vi "UPRcontroller_v00_basedonlsmv66.vi"() -> ()   [LabVIEW 2015] (continued)
                        n4652 = local read "Vx-ref"() -> (w1526:dbl)
                        n4653 = local read "Vy-ref"() -> (w1528:dbl)
                        n4654 = local read "avpp"() -> (w1527:i32)
                        n4655 = call "tt_timeandsamples.vi"("bin"=w1521, "refreshtime"=w1515, "srateAODOtt"=w1518, "tot#ofsamples"=w1523) -> ("refreshrate"=w1519:dbl, "refreshbuffer"=w1520:i32, "timetracecycles"=w1525:i32)  [unwired: 5 in]
                        n4656 = local read "bin"() -> (w1522:dbl)
                        n4657 = call "2pparameters.vi"("command"="get") -> ("params out"=w1534:T12)  [unwired: 1 in]
                        n4658 = Bundle By Name(cluster=w1534, "Drawing Mode"=w1507, "measpoints"=w1523, "tt_cycles"=w1525, "refreshbuffer"=w1520, "refreshrate"=w1519, "Vx-ref"=w1526, "Vy-ref"=w1528, "srate"=w1517, "finite"=w1530, "cont"=w1529, "wavdet"=w1531, "avpp"=w1527, "srateAODO"=w1524, "bufferAI"=w1520, "bin"=w1522, "Angle Img"=w1514, "Vxminref"=w1513, "Vxmaxref"=w1512, "Vyminref"=w1511, "Vymaxref"=w1510, "Xpixels Img"=w1509, "Ypixels Img"=w1508, "Pel"=w1506, "Vz-reset"=0.0, "AIoverride"=w1504, "type"="Timetrace") -> (w1532:T12)
                        n4659 = Reciprocal(x=w1519) -> (1/x=w1516:dbl)
                        n4660 = local write "refreshtime"(w1516) -> ()
                        n4661 = call "2pparameters.vi"("Params in"=w1532, "command"="set") -> ()  [unwired: 1 out]
                      }
                      frame "Lifetime (point)" {
                      }
                    }
                  }
                  frame #1 {
                    w1537 = FALSE ("wavdet")
                    n4662 = call "2pparameters.vi"("command"="get") -> ("params out"=w1541:T12)  [unwired: 1 in]
                    n4663 = Bundle By Name(cluster=w1541, "finite"=w1537, "cont"=w1537, "wavdet"=TRUE) -> (w1538:T12)
                    n4664 = call "2pparameters.vi"("Params in"=w1538, "command"="set") -> ()  [unwired: 1 out]
                  }
                  frame #2 {
                    n4665 = local read "Meastab"() -> (w1568:enum32{"X-Y Image", "Linescan", "Timetrace"})
                    n4666 = property on="AO channels" class="Ring (strict)"() -> ("RingText.Text"=w1543:string)  [unwired: 2 in, 2 out]
                    n4667 = property on="refwf" class="Ring (strict)"() -> ("RingText.Text"=w1567:string)  [unwired: 2 in, 2 out]
                    n4668 = local read "Build analog waveform tabs"() -> (w1566:enum32{"Square", "Triangle", "Matlab"})
                    n4669 = case shown="\"X-Y Image\", Default" w1568 {
                      tunnel: [w1574 w1575] -> w1565
                      frame "X-Y Image", Default {
                        n4670 = local read "Sampling rate"() -> (w1574:dbl)
                      }
                      frame "Timetrace" {
                        n4671 = local read "srateAODOtt"() -> (w1575:dbl)
                      }
                    }
                    n4672 = local read "Matlab waveform path"() -> (w1558:path)
                    n4673 = local read "Period (ms)"() -> (w1561:dbl)
                    n4674 = local read "Frequency"() -> (w1560:dbl)
                    n4675 = local read "Tri Repeats"() -> (w1559:dbl)
                    n4676 = local read "Repeats"() -> (w1564:dbl)
                    n4677 = local read "Cycles"() -> (w1563:dbl)
                    n4678 = local read "Pulses"() -> (w1562:dbl)
                    n4679 = call "matlabwfexistsdialogue.vi"("Matlab waveform path"=w1558) -> ("mtalab waveform path out"=w1557:path)
                    n4680 = call "wfsizecalc.vi"("Sampling frequency (Hz)"=w1565, "AOtab"=w1566, "reference waveforms to"=w1567, "channel"=w1543, "Repeats"=w1564, "Cycles"=w1563, "Matlab wave file"=w1557, "pulses"=w1562, "Period (ms)"=w1561, "Frequency"=w1560, "Tri Repeats"=w1559) -> ("total size GB"=w1552:dbl, "gigabytesize wf"=w1548:dbl)  [unwired: 3 in]
                    n4681 = Greater?(x=w1548, y=0.5) -> (0:w1549:bool)
                    n4682 = Number To Fractional String(number=w1548, width (-)=i16 3) -> (F-format string=w1554:string)  [unwired: 2 in]
                    n4683 = Number To Fractional String(number=w1552, width (-)=i16 4) -> (F-format string=w1553:string)  [unwired: 2 in]
                    n4684 = Concatenate Strings("this is a crude approximation:\nyou're about to create a  " ("message"), w1554, " GB waveform for a total of " ("string"), w1553, " GB. Are you sure?" ("string")) -> (w1550:string)
                    n4685 = case shown="True" w1549 {
                      tunnel: w1550 -> [_ w1573]
                      tunnel: [TRUE ("T button?") w1570] -> w1544
                      frame False {
                      }
                      frame True {
                        n4686 = Two Button Dialog(message=w1573, 1:"No, don't do this." ("Center Button Text (\"No\")"), 2:"Yes, continue. " ("Left Button Text (\"Yes\")")) -> (T button?=w1570:bool)
                      }
                    }
                  }
                  frame #3 {
                    n4687 = case shown="True" w1576 {
                      tunnel: [_ w1580] -> w1578
                      tunnel: [_ w1579] -> w1577
                      frame False {
                      }
                      frame True {
                        n4688 = local read "AO channels"() -> (w1582:u32)
                        n4689 = call "2pparameters.vi"("command"="get") -> ("params out"=w1584:T12)  [unwired: 1 in]
                        n4690 = Unbundle By Name(w1584) -> ("aAO"=w1583:u32[])
                        n4691 = Search 1D Array(1D array=w1583, element=w1582) -> (index of element=w1580:i32)  [unwired: 1 in]
                        n4692 = Greater?(x=w1580, y=-1) -> (0:w1579:bool)
                        n4693 = case shown="True" w1579 {
                          tunnel: w1580 -> [_ w1594]
                          frame False {
                          }
                          frame True {
                            n4694 = local read "Meastab"() -> (w1587:enum32{"X-Y Image", "Linescan", "Timetrace"})
                            n4695 = local read "Tri padding value"() -> (w1588:dbl)
                            n4696 = local read "Amplitude (V)"() -> (w1592:dbl)
                            n4697 = local read "Tri Phase (s)"() -> (w1589:dbl)
                            n4698 = local read "Tri Repeats"() -> (w1590:dbl)
                            n4699 = local read "Frequency"() -> (w1591:dbl)
                            n4700 = local read "Offset (V)"() -> (w1593:dbl)
                            n4701 = case shown="\"Timetrace\"" w1587 {
                              tunnel: [w1595 w1596] -> w1586
                              frame "X-Y Image", Default {
                                n4702 = local read "Sampling rate"() -> (w1595:dbl)
                              }
                              frame "Timetrace" {
                                n4703 = local read "srateAODOtt"() -> (w1596:dbl)
                              }
                            }
                            n4704 = call "replace AO tri wf param.vi"("padding value"=w1588, "index of AO wave"=w1594, "Tri phase"=w1589, "Sampling frequency (Hz)"=w1586, "Tri Repeats"=w1590, "Frequency"=w1591, "Amplitude (V)"=w1592, "Offset (V)"=w1593) -> ()
                          }
                        }
                      }
                    }
                  }
                  frame #4 {
                    n4705 = case shown="True" w1597 {
                      tunnel: w1599 -> [_ w1601]
                      tunnel: w1598 -> [_ w1600]
                      frame False {
                      }
                      frame True {
                        n4706 = case shown="True" w1600 {
                          tunnel: w1601 -> [_ w1610]
                          frame False {
                          }
                          frame True {
                            n4707 = call "waveformparamsv2.vi"("command"="get") -> ("Params out"=w1623:T17)  [unwired: 4 in, 2 out]
                            n4708 = Unbundle By Name(w1623) -> ("AO parameters"=w1622:T18)
                            n4709 = local read "Meastab"() -> (w1605:enum32{"X-Y Image", "Linescan", "Timetrace"})
                            n4710 = case shown="\"Timetrace\"" w1605 {
                              tunnel: [w1625 w1626] -> w1604
                              frame "X-Y Image", Default {
                                n4711 = local read "Sampling rate"() -> (w1625:dbl)
                              }
                              frame "Timetrace" {
                                n4712 = local read "srateAODOtt"() -> (w1626:dbl)
                              }
                            }
                            n4713 = Index Array(array=w1622, index=w1610) -> (element=w1612:T19)
                            n4714 = call "waveformsAObuffer.vi"("command"="get") -> ("AO wf out"=w1611:waveform(dbl)[])  [unwired: 1 in]
                            n4715 = call "generateTriWave_fromAOparameters.vi"("AO params"=w1612) -> ("Waveform"=w1609:waveform(dbl))  [unwired: 1 out]
                            n4716 = property on="refwf" class="Ring (strict)"() -> ("RingText.Text"=w1613:string)  [unwired: 2 in, 2 out]
                            n4717 = Replace Array Subset(array=w1611, new element=w1609, index=w1610) -> (w1608:waveform(dbl)[])
                            n4718 = call "waveformsDObuffer.vi"("command"="get") -> ("DO wf out"=w1618:digitalwaveform[])  [unwired: 1 in]
                            n4719 = call "correctwaveformsizetemp.vi"("new sampling frequency (Hz)"=w1604, "start"=FALSE, "reference waveforms to"=w1613, "Analog waveforms in"=w1608, "stop"=FALSE, "Digital waveforms in"=w1618) -> ("analog wf out"=w1616:waveform(dbl)[], "Digital wf out"=w1614:digitalwaveform[], "measpoints"=w1606:i32)
                            n4720 = local read "wavdet"() -> (w1607:bool)
                            n4721 = local write "Analog Lines Plot"(w1616) -> ()
                            n4722 = call "GetNumCamFramesv2.vi"("Digital Waveform Graph"=w1614) -> ("Numeric"=w1615:i32)  [unwired: 10 in]
                            n4723 = local write "Digital Lines Plot"(w1614) -> ()
                            n4724 = call "waveformsAObuffer.vi"("AO wf in"=w1616, "command"="set") -> ()  [unwired: 1 out]
                            n4725 = call "waveformsDObuffer.vi"("DO wf in"=w1614, "command"="set") -> ()  [unwired: 1 out]
                            n4726 = local write "Total Camera Frames"(w1615) -> ()
                            n4727 = case shown="True" w1607 {
                              tunnel: w1606 -> [_ w1627]
                              frame False {
                              }
                              frame True {
                                n4728 = local write "# of frames"(w1627) -> ()
                              }
                            }
                          }
                        }
                      }
                    }
                  }
                  frame #5 {
                    w1629 = FALSE ("addAO")
                    n4729 = case shown="True" w1628 {
                      frame False {
                      }
                      frame True {
                        n4730 = local write "not loadedtri"(FALSE ("not loadedtri")) -> ()
                      }
                    }
                    n4731 = local write "changeAOtri"(w1629) -> ()
                    n4732 = property on="load changed AOtri" class="Bool (strict)"("Val(Sgnl)"=w1629) -> ()  [unwired: 2 in, 2 out]
                    n4733 = local read "finite samples"() -> (w1630:bool)
                    n4734 = local read "continuous"() -> (w1631:bool)
                    n4735 = local read "wavdet"() -> (w1632:bool)
                    n4736 = call "2pparameters.vi"("command"="get") -> ("params out"=w1635:T12)  [unwired: 1 in]
                    n4737 = Bundle By Name(cluster=w1635, "finite"=w1630, "cont"=w1631, "wavdet"=w1632) -> (w1633:T12)
                    n4738 = call "2pparameters.vi"("Params in"=w1633, "command"="set") -> ()  [unwired: 1 out]
                  }
                }
              }
            }
          }
          event "Load Matlab Waveform": Value Change {
            n4739 = event-data() -> ("NewVal"=w1638:bool)  [unwired: 1 in, 5 out]
            n4740 = case shown="True" w1638 {
              frame False {
              }
              frame True {
                n4741 = stacked-sequence {
                  seq-local: [_ _ _ w1780 _ _] -> [_ _ _ _ w1798 _]
                  seq-local: [_ _ _ w1779 _ _] -> [_ _ _ _ w1797 _]
                  seq-local: [_ _ w1746 _ _ _] -> [_ _ _ w1778 w1796 w1827]
                  frame #0 {
                    n4742 = local read "Measurement"() -> (w1640:T4)
                    n4743 = case shown="\"X-Y-t movie\", Default" w1640 {
                      frame "X-Y-t movie", Default {
                        n4744 = local read "avpp"() -> (w1661:i32)
                        n4745 = local read "Angle ref"() -> (w1660:dbl)
                        n4746 = local read "ROI Type"() -> (w1659:u16)
                        n4747 = local read "xpixels ref"() -> (w1656:i32)
                        n4748 = local read "Vx-min ref"() -> (w1655:dbl)
                        n4749 = local read "Vx-max ref"() -> (w1654:dbl)
                        n4750 = local read "ypixels ref"() -> (w1652:i32)
                        n4751 = local read "Vy-min ref"() -> (w1653:dbl)
                        n4752 = local read "Vy-max ref"() -> (w1649:dbl)
                        n4753 = local read "Sampling rate"() -> (w1643:dbl)
                        n4754 = local read "finite samples"() -> (w1644:bool)
                        n4755 = local read "continuous"() -> (w1647:bool)
                        n4756 = local read "wavdet"() -> (w1648:bool)
                        n4757 = local read "# of frames"() -> (w1646:i32)
                        n4758 = local read "maxbufferAI"() -> (w1645:i32)
                        n4759 = local read "Override AI buffer"() -> (w1641:bool)
                        n4760 = call "2pparameters.vi"("command"="get") -> ("params out"=w1658:T12)  [unwired: 1 in]
                        n4761 = Bundle By Name(cluster=w1658, "type"="X-Y-t movie", "avpp"=w1661, "Angle Img"=w1660, "Xpixels Img"=w1656, "Vx-min Img"=w1655, "VX-max Img"=w1654, "Ypixels Img"=w1652, "Vy-min Img"=w1653, "Vy-max Img"=w1649, "srate"=w1643, "srate Img"=w1643, "finite"=w1644, "cont"=w1647, "wavdet"=w1648, "measpoints"=w1646, "maxbufferAI"=w1645, "Drawing Mode"=w1659, "Vz-reset"=0.0, "AIoverride"=w1641) -> (w1650:T12)
                        n4762 = call "2pparameters.vi"("Params in"=w1650, "command"="set") -> ()  [unwired: 1 out]
                      }
                      frame "X-Y-Z stack" {
                        n4763 = call "2pparameters.vi"("command"="get") -> ("params out"=w1665:T12)  [unwired: 1 in]
                        n4764 = Bundle By Name(cluster=w1665, "type"="X-Y-Z stack") -> (w1663:T12)
                        n4765 = call "2pparameters.vi"("Params in"=w1663, "command"="set") -> ()  [unwired: 1 out]
                      }
                      frame "Lifetime (scan)" {
                        n4766 = call "2pparameters.vi"("command"="get") -> ("params out"=w1670:T12)  [unwired: 1 in]
                        n4767 = Bundle By Name(cluster=w1670, "type"="Lifetime (scan)") -> (w1668:T12)
                        n4768 = call "2pparameters.vi"("Params in"=w1668, "command"="set") -> ()  [unwired: 1 out]
                      }
                      frame "Lifetime (contour)" {
                        n4769 = local read "Vy-min draw"() -> (w1680:dbl)
                        n4770 = local read "Vy-max draw"() -> (w1679:dbl)
                        n4771 = local read "Vx-min draw"() -> (w1682:dbl)
                        n4772 = local read "Vx-max draw"() -> (w1681:dbl)
                        n4773 = local read "xpixels ref"() -> (w1678:i32)
                        n4774 = local read "ypixels ref"() -> (w1677:i32)
                        n4775 = local read "ROI Type"() -> (w1676:u16)
                        n4776 = local read "srateAODOtt"() -> (w1687:dbl)
                        n4777 = local read "# of frames"() -> (w1692:i32)
                        n4778 = local read "refreshtime"() -> (w1684:dbl)
                        n4779 = local read "Pel"() -> (w1675:dbl)
                        n4780 = local read "bin"() -> (w1690:dbl)
                        n4781 = local read "Override AI buffer"() -> (w1673:bool)
                        n4782 = local read "finite samples"() -> (w1699:bool)
                        n4783 = local read "srateAODOtt"() -> (w1686:dbl)
                        n4784 = local read "srateAODOtt"() -> (w1693:dbl)
                        n4785 = local read "continuous"() -> (w1698:bool)
                        n4786 = local read "Angle ref"() -> (w1683:dbl)
                        n4787 = local read "wavdet"() -> (w1700:bool)
                        n4788 = local read "Vx-ref"() -> (w1695:dbl)
                        n4789 = local read "Vy-ref"() -> (w1697:dbl)
                        n4790 = local read "avpp"() -> (w1696:i32)
                        n4791 = call "tt_timeandsamples.vi"("bin"=w1690, "refreshtime"=w1684, "srateAODOtt"=w1687, "tot#ofsamples"=w1692) -> ("refreshrate"=w1688:dbl, "refreshbuffer"=w1689:i32, "timetracecycles"=w1694:i32)  [unwired: 5 in]
                        n4792 = local read "bin"() -> (w1691:dbl)
                        n4793 = call "2pparameters.vi"("command"="get") -> ("params out"=w1703:T12)  [unwired: 1 in]
                        n4794 = Bundle By Name(cluster=w1703, "Drawing Mode"=w1676, "measpoints"=w1692, "tt_cycles"=w1694, "refreshbuffer"=w1689, "refreshrate"=w1688, "Vx-ref"=w1695, "Vy-ref"=w1697, "srate"=w1686, "finite"=w1699, "cont"=w1698, "wavdet"=w1700, "avpp"=w1696, "srateAODO"=w1693, "bufferAI"=w1689, "bin"=w1691, "Angle Img"=w1683, "Vxminref"=w1682, "Vxmaxref"=w1681, "Vyminref"=w1680, "Vymaxref"=w1679, "Xpixels Img"=w1678, "Ypixels Img"=w1677, "Pel"=w1675, "Vz-reset"=0.0, "AIoverride"=w1673, "type"="Lifetime (contour)") -> (w1701:T12)
                        n4795 = Reciprocal(x=w1688) -> (1/x=w1685:dbl)
                        n4796 = local write "refreshtime"(w1685) -> ()
                        n4797 = call "2pparameters.vi"("Params in"=w1701, "command"="set") -> ()  [unwired: 1 out]
                      }
                      frame "X-Y-Z-t movie" {
                      }
                      frame "linescan" {
                      }
                      frame "Timetrace" {
                        n4798 = local read "Vy-min draw"() -> (w1713:dbl)
                        n4799 = local read "Vy-max draw"() -> (w1712:dbl)
                        n4800 = local read "Vx-min draw"() -> (w1715:dbl)
                        n4801 = local read "Vx-max draw"() -> (w1714:dbl)
                        n4802 = local read "xpixels ref"() -> (w1711:i32)
                        n4803 = local read "ypixels ref"() -> (w1710:i32)
                        n4804 = local read "ROI Type"() -> (w1709:u16)
                        n4805 = local read "srateAODOtt"() -> (w1720:dbl)
                        n4806 = local read "# of frames"() -> (w1725:i32)
                        n4807 = local read "refreshtime"() -> (w1717:dbl)
                        n4808 = local read "Pel"() -> (w1708:dbl)
                        n4809 = local read "bin"() -> (w1723:dbl)
                        n4810 = local read "Override AI buffer"() -> (w1706:bool)
                        n4811 = local read "finite samples"() -> (w1732:bool)
                        n4812 = local read "srateAODOtt"() -> (w1719:dbl)
                        n4813 = local read "srateAODOtt"() -> (w1726:dbl)
                        n4814 = local read "continuous"() -> (w1731:bool)
                        n4815 = local read "Angle ref"() -> (w1716:dbl)
                        n4816 = local read "wavdet"() -> (w1733:bool)
                        n4817 = local read "Vx-ref"() -> (w1728:dbl)
                        n4818 = local read "Vy-ref"() -> (w1730:dbl)
                        n4819 = local read "avpp"() -> (w1729:i32)
                        n4820 = call "tt_timeandsamples.vi"("bin"=w1723, "refreshtime"=w1717, "srateAODOtt"=w1720, "tot#ofsamples"=w1725) -> ("refreshrate"=w1721:dbl, "refreshbuffer"=w1722:i32, "timetracecycles"=w1727:i32)  [unwired: 5 in]
                        n4821 = local read "bin"() -> (w1724:dbl)
                        n4822 = call "2pparameters.vi"("command"="get") -> ("params out"=w1736:T12)  [unwired: 1 in]
                        n4823 = Bundle By Name(cluster=w1736, "Drawing Mode"=w1709, "measpoints"=w1725, "tt_cycles"=w1727, "refreshbuffer"=w1722, "refreshrate"=w1721, "Vx-ref"=w1728, "Vy-ref"=w1730, "srate"=w1719, "finite"=w1732, "cont"=w1731, "wavdet"=w1733, "avpp"=w1729, "srateAODO"=w1726, "bufferAI"=w1722, "bin"=w1724, "Angle Img"=w1716, "Vxminref"=w1715, "Vxmaxref"=w1714, "Vyminref"=w1713, "Vymaxref"=w1712, "Xpixels Img"=w1711, "Ypixels Img"=w1710, "Pel"=w1708, "Vz-reset"=0.0, "AIoverride"=w1706, "type"="Timetrace") -> (w1734:T12)
                        n4824 = Reciprocal(x=w1721) -> (1/x=w1718:dbl)
                        n4825 = local write "refreshtime"(w1718) -> ()
                        n4826 = call "2pparameters.vi"("Params in"=w1734, "command"="set") -> ()  [unwired: 1 out]
                      }
                      frame "Lifetime (point)" {
                      }
                    }
                    n4827 = local write "changeAOmatlab"(TRUE ("addAO")) -> ()
                  }
                  frame #1 {
                    w1739 = FALSE ("wavdet")
                    n4828 = call "2pparameters.vi"("command"="get") -> ("params out"=w1743:T12)  [unwired: 1 in]
                    n4829 = Bundle By Name(cluster=w1743, "finite"=w1739, "cont"=w1739, "wavdet"=TRUE) -> (w1740:T12)
                    n4830 = call "2pparameters.vi"("Params in"=w1740, "command"="set") -> ()  [unwired: 1 out]
                  }
                  frame #2 {
                    n4831 = local read "Meastab"() -> (w1770:enum32{"X-Y Image", "Linescan", "Timetrace"})
                    n4832 = property on="AO channels" class="Ring (strict)"() -> ("RingText.Text"=w1745:string)  [unwired: 2 in, 2 out]
                    n4833 = property on="refwf" class="Ring (strict)"() -> ("RingText.Text"=w1769:string)  [unwired: 2 in, 2 out]
                    n4834 = local read "Build analog waveform tabs"() -> (w1768:enum32{"Square", "Triangle", "Matlab"})
                    n4835 = case shown="\"X-Y Image\", Default" w1770 {
                      tunnel: [w1776 w1777] -> w1767
                      frame "X-Y Image", Default {
                        n4836 = local read "Sampling rate"() -> (w1776:dbl)
                      }
                      frame "Timetrace" {
                        n4837 = local read "srateAODOtt"() -> (w1777:dbl)
                      }
                    }
                    n4838 = local read "Matlab waveform path"() -> (w1760:path)
                    n4839 = local read "Period (ms)"() -> (w1763:dbl)
                    n4840 = local read "Frequency"() -> (w1762:dbl)
                    n4841 = local read "Tri Repeats"() -> (w1761:dbl)
                    n4842 = local read "Repeats"() -> (w1766:dbl)
                    n4843 = local read "Cycles"() -> (w1765:dbl)
                    n4844 = local read "Pulses"() -> (w1764:dbl)
                    n4845 = call "matlabwfexistsdialogue.vi"("Matlab waveform path"=w1760) -> ("mtalab waveform path out"=w1759:path)
                    n4846 = call "wfsizecalc.vi"("Sampling frequency (Hz)"=w1767, "AOtab"=w1768, "reference waveforms to"=w1769, "channel"=w1745, "Repeats"=w1766, "Cycles"=w1765, "Matlab wave file"=w1759, "pulses"=w1764, "Period (ms)"=w1763, "Frequency"=w1762, "Tri Repeats"=w1761) -> ("total size GB"=w1754:dbl, "gigabytesize wf"=w1750:dbl)  [unwired: 3 in]
                    n4847 = Greater?(x=w1750, y=0.5) -> (0:w1751:bool)
                    n4848 = Number To Fractional String(number=w1750, width (-)=i16 3) -> (F-format string=w1756:string)  [unwired: 2 in]
                    n4849 = Number To Fractional String(number=w1754, width (-)=i16 4) -> (F-format string=w1755:string)  [unwired: 2 in]
                    n4850 = Concatenate Strings("this is a crude approximation:\nyou're about to create a  " ("message"), w1756, " GB waveform for a total of " ("string"), w1755, " GB. Are you sure?" ("string")) -> (w1752:string)
                    n4851 = case shown="True" w1751 {
                      tunnel: w1752 -> [_ w1775]
                      tunnel: [TRUE ("T button?") w1772] -> w1746
                      frame False {
                      }
                      frame True {
                        n4852 = Two Button Dialog(message=w1775, 1:"No, don't do this." ("Center Button Text (\"No\")"), 2:"Yes, continue. " ("Left Button Text (\"Yes\")")) -> (T button?=w1772:bool)
                      }
                    }
                  }
                  frame #3 {
                    n4853 = case shown="True" w1778 {
                      tunnel: [_ w1782] -> w1780
                      tunnel: [_ w1781] -> w1779
                      frame False {
                      }
                      frame True {
                        n4854 = local read "AO channels"() -> (w1784:u32)
                        n4855 = call "2pparameters.vi"("command"="get") -> ("params out"=w1786:T12)  [unwired: 1 in]
                        n4856 = Unbundle By Name(w1786) -> ("aAO"=w1785:u32[])
                        n4857 = Search 1D Array(1D array=w1785, element=w1784) -> (index of element=w1782:i32)  [unwired: 1 in]
                        n4858 = Greater?(x=w1782, y=-1) -> (0:w1781:bool)
                        n4859 = case shown="True" w1781 {
                          tunnel: w1782 -> [_ w1793]
                          frame False {
                          }
                          frame True {
                            n4860 = local read "Meastab"() -> (w1789:enum32{"X-Y Image", "Linescan", "Timetrace"})
                            n4861 = local read "Matlab waveform path"() -> (w1791:path)
                            n4862 = local read "Matlab padding value"() -> (w1792:dbl)
                            n4863 = case shown="\"Timetrace\"" w1789 {
                              tunnel: [w1794 w1795] -> w1788
                              frame "X-Y Image", Default {
                                n4864 = local read "Sampling rate"() -> (w1794:dbl)
                              }
                              frame "Timetrace" {
                                n4865 = local read "srateAODOtt"() -> (w1795:dbl)
                              }
                            }
                            n4866 = call "matlabwfexistsdialogue.vi"("Matlab waveform path"=w1791) -> ("mtalab waveform path out"=w1790:path)
                            n4867 = call "replace AO matlab param.vi"("Sampling frequency (Hz)"=w1788, "matlab wave file"=w1790, "index of AO wave"=w1793, "padding value"=w1792) -> ()  [unwired: 7 in]
                          }
                        }
                      }
                    }
                  }
                  frame #4 {
                    n4868 = case shown="True" w1796 {
                      tunnel: w1798 -> [_ w1800]
                      tunnel: w1797 -> [_ w1799]
                      frame False {
                      }
                      frame True {
                        n4869 = case shown="True" w1799 {
                          tunnel: w1800 -> [_ w1807]
                          frame False {
                          }
                          frame True {
                            n4870 = local read "Meastab"() -> (w1804:enum32{"X-Y Image", "Linescan", "Timetrace"})
                            n4871 = call "waveformparamsv2.vi"("command"="get") -> ("Params out"=w1810:T17)  [unwired: 4 in, 2 out]
                            n4872 = Unbundle By Name(w1810) -> ("AO parameters"=w1809:T18)
                            n4873 = case shown="\"Timetrace\"" w1804 {
                              tunnel: [w1824 w1825] -> w1803
                              frame "X-Y Image", Default {
                                n4874 = local read "Sampling rate"() -> (w1824:dbl)
                              }
                              frame "Timetrace" {
                                n4875 = local read "srateAODOtt"() -> (w1825:dbl)
                              }
                            }
                            n4876 = Index Array(array=w1809, index=w1807) -> (element=w1808:T19)
                            n4877 = call "waveformsAObuffer.vi"("command"="get") -> ("AO wf out"=w1814:waveform(dbl)[])  [unwired: 1 in]
                            n4878 = call "matlabAOwffromparam.vi"("Cluster"=w1808) -> ("Waveform"=w1812:waveform(dbl))  [unwired: 1 out]
                            n4879 = property on="refwf" class="Ring (strict)"() -> ("RingText.Text"=w1815:string)  [unwired: 2 in, 2 out]
                            n4880 = Replace Array Subset(array=w1814, new element=w1812, index=w1807) -> (w1813:waveform(dbl)[])
                            n4881 = call "waveformsDObuffer.vi"("command"="get") -> ("DO wf out"=w1820:digitalwaveform[])  [unwired: 1 in]
                            n4882 = call "correctwaveformsizetemp.vi"("new sampling frequency (Hz)"=w1803, "start"=FALSE, "reference waveforms to"=w1815, "Analog waveforms in"=w1813, "stop"=FALSE, "Digital waveforms in"=w1820) -> ("analog wf out"=w1818:waveform(dbl)[], "Digital wf out"=w1816:digitalwaveform[], "measpoints"=w1805:i32)
                            n4883 = local read "wavdet"() -> (w1806:bool)
                            n4884 = local write "Analog Lines Plot"(w1818) -> ()
                            n4885 = call "GetNumCamFramesv2.vi"("Digital Waveform Graph"=w1816) -> ("Numeric"=w1817:i32)  [unwired: 10 in]
                            n4886 = local write "Digital Lines Plot"(w1816) -> ()
                            n4887 = call "waveformsAObuffer.vi"("AO wf in"=w1818, "command"="set") -> ()  [unwired: 1 out]
                            n4888 = call "waveformsDObuffer.vi"("DO wf in"=w1816, "command"="set") -> ()  [unwired: 1 out]
                            n4889 = local write "Total Camera Frames"(w1817) -> ()
                            n4890 = case shown="True" w1806 {
                              tunnel: w1805 -> [_ w1826]
                              frame False {
                              }
                              frame True {
                                n4891 = local write "# of frames"(w1826) -> ()
                              }
                            }
                          }
                        }
                      }
                    }
                  }
                  frame #5 {
                    w1828 = FALSE ("addAO")
                    n4892 = case shown="True" w1827 {
                      frame False {
                      }
                      frame True {
                        n4893 = local write "not loadedml"(FALSE ("not loadedml")) -> ()
                      }
                    }
                    n4894 = local read "finite samples"() -> (w1829:bool)
                    n4895 = local read "continuous"() -> (w1830:bool)
                    n4896 = local read "wavdet"() -> (w1831:bool)
                    n4897 = property on="Load Matlab Waveform" class="Bool (strict)"("Val(Sgnl)"=w1828) -> ()  [unwired: 2 in, 2 out]
                    n4898 = local write "changeAOmatlab"(w1828) -> ()
                    n4899 = call "2pparameters.vi"("command"="get") -> ("params out"=w1834:T12)  [unwired: 1 in]
                    n4900 = Bundle By Name(cluster=w1834, "finite"=w1829, "cont"=w1830, "wavdet"=w1831) -> (w1832:T12)
                    n4901 = call "2pparameters.vi"("Params in"=w1832, "command"="set") -> ()  [unwired: 1 out]
                  }
                }
              }
            }
          }
          event "Load Matlab Waveform DO": Value Change {
            n4902 = event-data() -> ("NewVal"=w1837:bool)  [unwired: 1 in, 5 out]
            n4903 = case shown="True" w1837 {
              frame False {
              }
              frame True {
                n4904 = stacked-sequence {
                  seq-local: [_ _ w1945 _ _] -> [_ _ _ w1960 _]
                  seq-local: [_ _ w1944 _ _] -> [_ _ _ w1959 _]
                  frame #0 {
                    n4905 = local read "Measurement"() -> (w1839:T4)
                    n4906 = case shown="\"X-Y-t movie\", Default" w1839 {
                      frame "X-Y-t movie", Default {
                        n4907 = local read "avpp"() -> (w1860:i32)
                        n4908 = local read "Angle ref"() -> (w1859:dbl)
                        n4909 = local read "ROI Type"() -> (w1858:u16)
                        n4910 = local read "xpixels ref"() -> (w1855:i32)
                        n4911 = local read "Vx-min ref"() -> (w1854:dbl)
                        n4912 = local read "Vx-max ref"() -> (w1853:dbl)
                        n4913 = local read "ypixels ref"() -> (w1851:i32)
                        n4914 = local read "Vy-min ref"() -> (w1852:dbl)
                        n4915 = local read "Vy-max ref"() -> (w1848:dbl)
                        n4916 = local read "Sampling rate"() -> (w1842:dbl)
                        n4917 = local read "finite samples"() -> (w1843:bool)
                        n4918 = local read "continuous"() -> (w1846:bool)
                        n4919 = local read "wavdet"() -> (w1847:bool)
                        n4920 = local read "# of frames"() -> (w1845:i32)
                        n4921 = local read "maxbufferAI"() -> (w1844:i32)
                        n4922 = local read "Override AI buffer"() -> (w1840:bool)
                        n4923 = call "2pparameters.vi"("command"="get") -> ("params out"=w1857:T12)  [unwired: 1 in]
                        n4924 = Bundle By Name(cluster=w1857, "type"="X-Y-t movie", "avpp"=w1860, "Angle Img"=w1859, "Xpixels Img"=w1855, "Vx-min Img"=w1854, "VX-max Img"=w1853, "Ypixels Img"=w1851, "Vy-min Img"=w1852, "Vy-max Img"=w1848, "srate"=w1842, "srate Img"=w1842, "finite"=w1843, "cont"=w1846, "wavdet"=w1847, "measpoints"=w1845, "maxbufferAI"=w1844, "Drawing Mode"=w1858, "Vz-reset"=0.0, "AIoverride"=w1840) -> (w1849:T12)
                        n4925 = call "2pparameters.vi"("Params in"=w1849, "command"="set") -> ()  [unwired: 1 out]
                      }
                      frame "X-Y-Z stack" {
                        n4926 = call "2pparameters.vi"("command"="get") -> ("params out"=w1864:T12)  [unwired: 1 in]
                        n4927 = Bundle By Name(cluster=w1864, "type"="X-Y-Z stack") -> (w1862:T12)
                        n4928 = call "2pparameters.vi"("Params in"=w1862, "command"="set") -> ()  [unwired: 1 out]
                      }
                      frame "Lifetime (scan)" {
                        n4929 = call "2pparameters.vi"("command"="get") -> ("params out"=w1869:T12)  [unwired: 1 in]
                        n4930 = Bundle By Name(cluster=w1869, "type"="Lifetime (scan)") -> (w1867:T12)
                        n4931 = call "2pparameters.vi"("Params in"=w1867, "command"="set") -> ()  [unwired: 1 out]
                      }
                      frame "Lifetime (contour)" {
                        n4932 = local read "Vy-min draw"() -> (w1879:dbl)
                        n4933 = local read "Vy-max draw"() -> (w1878:dbl)
                        n4934 = local read "Vx-min draw"() -> (w1881:dbl)
                        n4935 = local read "Vx-max draw"() -> (w1880:dbl)
                        n4936 = local read "xpixels ref"() -> (w1877:i32)
                        n4937 = local read "ypixels ref"() -> (w1876:i32)
                        n4938 = local read "ROI Type"() -> (w1875:u16)
                        n4939 = local read "srateAODOtt"() -> (w1886:dbl)
                        n4940 = local read "# of frames"() -> (w1891:i32)
                        n4941 = local read "refreshtime"() -> (w1883:dbl)
                        n4942 = local read "Pel"() -> (w1874:dbl)
                        n4943 = local read "bin"() -> (w1889:dbl)
                        n4944 = local read "Override AI buffer"() -> (w1872:bool)
                        n4945 = local read "finite samples"() -> (w1898:bool)
                        n4946 = local read "srateAODOtt"() -> (w1885:dbl)
                        n4947 = local read "srateAODOtt"() -> (w1892:dbl)
                        n4948 = local read "continuous"() -> (w1897:bool)
                        n4949 = local read "Angle ref"() -> (w1882:dbl)
                        n4950 = local read "wavdet"() -> (w1899:bool)
                        n4951 = local read "Vx-ref"() -> (w1894:dbl)
                        n4952 = local read "Vy-ref"() -> (w1896:dbl)
                        n4953 = local read "avpp"() -> (w1895:i32)
                        n4954 = call "tt_timeandsamples.vi"("bin"=w1889, "refreshtime"=w1883, "srateAODOtt"=w1886, "tot#ofsamples"=w1891) -> ("refreshrate"=w1887:dbl, "refreshbuffer"=w1888:i32, "timetracecycles"=w1893:i32)  [unwired: 5 in]
                        n4955 = local read "bin"() -> (w1890:dbl)
                        n4956 = call "2pparameters.vi"("command"="get") -> ("params out"=w1902:T12)  [unwired: 1 in]
                        n4957 = Bundle By Name(cluster=w1902, "Drawing Mode"=w1875, "measpoints"=w1891, "tt_cycles"=w1893, "refreshbuffer"=w1888, "refreshrate"=w1887, "Vx-ref"=w1894, "Vy-ref"=w1896, "srate"=w1885, "finite"=w1898, "cont"=w1897, "wavdet"=w1899, "avpp"=w1895, "srateAODO"=w1892, "bufferAI"=w1888, "bin"=w1890, "Angle Img"=w1882, "Vxminref"=w1881, "Vxmaxref"=w1880, "Vyminref"=w1879, "Vymaxref"=w1878, "Xpixels Img"=w1877, "Ypixels Img"=w1876, "Pel"=w1874, "Vz-reset"=0.0, "AIoverride"=w1872, "type"="Lifetime (contour)") -> (w1900:T12)
                        n4958 = Reciprocal(x=w1887) -> (1/x=w1884:dbl)
                        n4959 = local write "refreshtime"(w1884) -> ()
                        n4960 = call "2pparameters.vi"("Params in"=w1900, "command"="set") -> ()  [unwired: 1 out]
                      }
                      frame "X-Y-Z-t movie" {
                      }
                      frame "linescan" {
                      }
                      frame "Timetrace" {
                        n4961 = local read "Vy-min draw"() -> (w1912:dbl)
                        n4962 = local read "Vy-max draw"() -> (w1911:dbl)
                        n4963 = local read "Vx-min draw"() -> (w1914:dbl)
                        n4964 = local read "Vx-max draw"() -> (w1913:dbl)
                        n4965 = local read "xpixels ref"() -> (w1910:i32)
                        n4966 = local read "ypixels ref"() -> (w1909:i32)
                        n4967 = local read "ROI Type"() -> (w1908:u16)
                        n4968 = local read "srateAODOtt"() -> (w1919:dbl)
                        n4969 = local read "# of frames"() -> (w1924:i32)
                        n4970 = local read "refreshtime"() -> (w1916:dbl)
                        n4971 = local read "Pel"() -> (w1907:dbl)
                        n4972 = local read "bin"() -> (w1922:dbl)
                        n4973 = local read "Override AI buffer"() -> (w1905:bool)
                        n4974 = local read "finite samples"() -> (w1931:bool)
                        n4975 = local read "srateAODOtt"() -> (w1918:dbl)
                        n4976 = local read "srateAODOtt"() -> (w1925:dbl)
                        n4977 = local read "continuous"() -> (w1930:bool)
                        n4978 = local read "Angle ref"() -> (w1915:dbl)
                        n4979 = local read "wavdet"() -> (w1932:bool)
                        n4980 = local read "Vx-ref"() -> (w1927:dbl)
                        n4981 = local read "Vy-ref"() -> (w1929:dbl)
                        n4982 = local read "avpp"() -> (w1928:i32)
                        n4983 = call "tt_timeandsamples.vi"("bin"=w1922, "refreshtime"=w1916, "srateAODOtt"=w1919, "tot#ofsamples"=w1924) -> ("refreshrate"=w1920:dbl, "refreshbuffer"=w1921:i32, "timetracecycles"=w1926:i32)  [unwired: 5 in]
                        n4984 = local read "bin"() -> (w1923:dbl)
                        n4985 = call "2pparameters.vi"("command"="get") -> ("params out"=w1935:T12)  [unwired: 1 in]
                        n4986 = Bundle By Name(cluster=w1935, "Drawing Mode"=w1908, "measpoints"=w1924, "tt_cycles"=w1926, "refreshbuffer"=w1921, "refreshrate"=w1920, "Vx-ref"=w1927, "Vy-ref"=w1929, "srate"=w1918, "finite"=w1931, "cont"=w1930, "wavdet"=w1932, "avpp"=w1928, "srateAODO"=w1925, "bufferAI"=w1921, "bin"=w1923, "Angle Img"=w1915, "Vxminref"=w1914, "Vxmaxref"=w1913, "Vyminref"=w1912, "Vymaxref"=w1911, "Xpixels Img"=w1910, "Ypixels Img"=w1909, "Pel"=w1907, "Vz-reset"=0.0, "AIoverride"=w1905, "type"="Timetrace") -> (w1933:T12)
                        n4987 = Reciprocal(x=w1920) -> (1/x=w1917:dbl)
                        n4988 = local write "refreshtime"(w1917) -> ()
                        n4989 = call "2pparameters.vi"("Params in"=w1933, "command"="set") -> ()  [unwired: 1 out]
                      }
                      frame "Lifetime (point)" {
                      }
                    }
                    n4990 = local write "changeDOmatlab"(TRUE ("addAO")) -> ()
                  }
                  frame #1 {
                    w1938 = FALSE ("wavdet")
                    n4991 = call "2pparameters.vi"("command"="get") -> ("params out"=w1942:T12)  [unwired: 1 in]
                    n4992 = Bundle By Name(cluster=w1942, "finite"=w1938, "cont"=w1938, "wavdet"=TRUE) -> (w1939:T12)
                    n4993 = call "2pparameters.vi"("Params in"=w1939, "command"="set") -> ()  [unwired: 1 out]
                  }
                  frame #2 {
                    n4994 = local read "DO channels"() -> (w1947:u16)
                    n4995 = call "2pparameters.vi"("command"="get") -> ("params out"=w1949:T12)  [unwired: 1 in]
                    n4996 = Unbundle By Name(w1949) -> ("aDO"=w1948:u32[])
                    n4997 = Search 1D Array(1D array=w1948, element=w1947) -> (index of element=w1945:i32)  [unwired: 1 in]
                    n4998 = Greater?(x=w1945, y=-1) -> (0:w1944:bool)
                    n4999 = case shown="True" w1944 {
                      tunnel: w1945 -> [_ w1956]
                      frame False {
                      }
                      frame True {
                        n5000 = local read "Meastab"() -> (w1952:enum32{"X-Y Image", "Linescan", "Timetrace"})
                        n5001 = local read "Matlab waveform path DO"() -> (w1954:path)
                        n5002 = local read "Matlab padding value DO"() -> (w1955:dbl)
                        n5003 = case shown="\"Timetrace\"" w1952 {
                          tunnel: [w1957 w1958] -> w1951
                          frame "X-Y Image", Default {
                            n5004 = local read "Sampling rate"() -> (w1957:dbl)
                          }
                          frame "Timetrace" {
                            n5005 = local read "srateAODOtt"() -> (w1958:dbl)
                          }
                        }
                        n5006 = call "matlabwfexistsdialogue.vi"("Matlab waveform path"=w1954) -> ("mtalab waveform path out"=w1953:path)
                        n5007 = call "replace DO matlab param.vi"("Sampling frequency (Hz)"=w1951, "matlab wave number"=w1953, "index of DO wave"=w1956, "padding value"=w1955) -> ()  [unwired: 7 in]
                      }
                    }
                  }
                  frame #3 {
                    n5008 = case shown="True" w1959 {
                      tunnel: w1960 -> [_ w1969]
                      frame False {
                      }
                      frame True {
                        n5009 = local read "Meastab"() -> (w1964:enum32{"X-Y Image", "Linescan", "Timetrace"})
                        n5010 = call "waveformparamsv2.vi"("command"="get") -> ("Params out"=w1982:T17)  [unwired: 4 in, 2 out]
                        n5011 = Unbundle By Name(w1982) -> ("DO parameters"=w1981:T20)
                        n5012 = case shown="\"Timetrace\"" w1964 {
                          tunnel: [w1984 w1985] -> w1963
                          frame "X-Y Image", Default {
                            n5013 = local read "Sampling rate"() -> (w1984:dbl)
                          }
                          frame "Timetrace" {
                            n5014 = local read "srateAODOtt"() -> (w1985:dbl)
                          }
                        }
                        n5015 = Index Array(array=w1981, index=w1969) -> (element=w1968:T21)
                        n5016 = call "waveformsDObuffer.vi"("command"="get") -> ("DO wf out"=w1979:digitalwaveform[])  [unwired: 1 in]
                        n5017 = property on="refwf" class="Ring (strict)"() -> ("RingText.Text"=w1971:string)  [unwired: 2 in, 2 out]
                        n5018 = call "matlabDOwffromparam.vi"("waveform params"=w1968) -> ("digital waveform"=w1967:digitalwaveform)
                        n5019 = Replace Array Subset(array=w1979, new element=w1967, index=w1969) -> (w1970:digitalwaveform[])
                        n5020 = call "waveformsAObuffer.vi"("command"="get") -> ("AO wf out"=w1978:waveform(dbl)[])  [unwired: 1 in]
                        n5021 = local read "wavdet"() -> (w1966:bool)
                        n5022 = call "correctwaveformsizetemp.vi"("new sampling frequency (Hz)"=w1963, "start"=FALSE, "reference waveforms to"=w1971, "Analog waveforms in"=w1978, "stop"=FALSE, "Digital waveforms in"=w1970) -> ("analog wf out"=w1974:waveform(dbl)[], "Digital wf out"=w1972:digitalwaveform[], "measpoints"=w1965:i32)
                        n5023 = local write "Analog Lines Plot"(w1974) -> ()
                        n5024 = call "GetNumCamFramesv2.vi"("Digital Waveform Graph"=w1972) -> ("Numeric"=w1973:i32)  [unwired: 10 in]
                        n5025 = local write "Digital Lines Plot"(w1972) -> ()
                        n5026 = case shown="True" w1966 {
                          tunnel: w1965 -> [_ w1986]
                          frame False {
                          }
                          frame True {
                            n5027 = local write "# of frames"(w1986) -> ()
                          }
                        }
                        n5028 = call "waveformsAObuffer.vi"("AO wf in"=w1974, "command"="set") -> ()  [unwired: 1 out]
                        n5029 = call "waveformsDObuffer.vi"("DO wf in"=w1972, "command"="set") -> ()  [unwired: 1 out]
                        n5030 = local write "Total Camera Frames"(w1973) -> ()
                      }
                    }
                  }
                  frame #4 {
                    w1988 = FALSE ("addAO")
                    n5031 = local read "finite samples"() -> (w1989:bool)
                    n5032 = local read "continuous"() -> (w1990:bool)
                    n5033 = local read "wavdet"() -> (w1991:bool)
                    n5034 = call "2pparameters.vi"("command"="get") -> ("params out"=w1994:T12)  [unwired: 1 in]
                    n5035 = Bundle By Name(cluster=w1994, "finite"=w1989, "cont"=w1990, "wavdet"=w1991) -> (w1992:T12)
                    n5036 = local write "not loadedDOml"(FALSE ("not loadedDO")) -> ()
                    n5037 = local write "changeDOmatlab"(w1988) -> ()
                    n5038 = property on="Load Matlab Waveform DO" class="Bool (strict)"("Val(Sgnl)"=w1988) -> ()  [unwired: 2 in, 2 out]
                    n5039 = call "2pparameters.vi"("Params in"=w1992, "command"="set") -> ()  [unwired: 1 out]
                  }
                }
              }
            }
          }
          event "Add settings": Value Change {
            n5040 = event-data() -> ("NewVal"=w1996:bool)  [unwired: 1 in, 5 out]
            n5041 = case shown="True" w1996 {
              frame False {
              }
              frame True {
                n5042 = stacked-sequence {
                  frame #0 {
                    n5043 = call "wfsettings.vi"("command"="get") -> ("wfsettings out"=w1999:T30)  [unwired: 2 in, 1 out]
                    n5044 = in-place {
                      n5045 = in-place-cluster #53(w1999) -> ("settings names"=w2004:string[], "settings locations"=w2006:path[])
                      n5046 = local read "Setting location"() -> (w2002:path)
                      n5047 = local read "Nickname"() -> (w2001:string)
                      n5048 = Build Array (concatenate)(w2004, w2001) -> (w2003:string[])
                      n5049 = property on="Loaded settings" class="Ring (strict)"("Strings []"=w2003) -> ()  [unwired: 2 in, 2 out]
                      n5050 = Build Array (concatenate)(w2006, w2002) -> (w2005:path[])
                      n5051 = in-place-cluster #53("settings names"=w2003, "settings locations"=w2005) -> (w1997:T30)
                    }
                    n5052 = call "wfsettings.vi"("wfsettings in"=w1997, "command"="set") -> ()  [unwired: 1 in, 2 out]
                  }
                  frame #1 {
                    n5053 = property on="Add settings" class="Bool (strict)"("Val(Sgnl)"=FALSE ("Value (Signaling)")) -> ()  [unwired: 2 in, 2 out]
                  }
                }
              }
            }
          }
          event "Rem setting": Value Change {
            n5054 = event-data() -> ("NewVal"=w2008:bool)  [unwired: 1 in, 5 out]
            n5055 = case shown="True" w2008 {
              frame False {
              }
              frame True {
                n5056 = stacked-sequence {
                  frame #0 {
                    n5057 = call "wfsettings.vi"("command"="get") -> ("wfsettings out"=w2011:T30)  [unwired: 2 in, 1 out]
                    n5058 = in-place {
                      n5059 = in-place-cluster #54(w2011) -> ("settings names"=w2016:string[], "settings locations"=w2014:path[])
                      n5060 = property on="Loaded settings" class="Ring (strict)"() -> ("RingText.Text"=w2017:string)  [unwired: 2 in, 2 out]
                      n5061 = Search 1D Array(1D array=w2016, element=w2017) -> (index of element=w2018:i32)  [unwired: 1 in]
                      n5062 = Delete From Array(array=w2016, index=w2018) -> (array with subset deleted=w2015:string[])  [unwired: 1 in, 1 out]
                      n5063 = Delete From Array(array=w2014, index=w2018) -> (array with subset deleted=w2013:path[])  [unwired: 1 in, 1 out]
                      n5064 = property on="Loaded settings" class="Ring (strict)"("Strings []"=w2015) -> ()  [unwired: 2 in, 2 out]
                      n5065 = in-place-cluster #54("settings names"=w2015, "settings locations"=w2013) -> (w2009:T30)
                    }
                    n5066 = call "wfsettings.vi"("wfsettings in"=w2009, "command"="set") -> ()  [unwired: 1 in, 2 out]
                  }
                  frame #1 {
                    n5067 = property on="Rem setting" class="Bool (strict)"("Val(Sgnl)"=FALSE ("Value (Signaling)")) -> ()  [unwired: 2 in, 2 out]
                  }
                }
              }
            }
          }
          event "Update settings": Value Change {
            n5068 = event-data() -> ("NewVal"=w2020:bool)  [unwired: 1 in, 5 out]
            n5069 = case shown="True" w2020 {
              frame False {
              }
              frame True {
                n5070 = stacked-sequence {
                  frame #0 {
                    n5071 = local read "Measurement"() -> (w2021:T4)
                    n5072 = case shown="\"X-Y-t movie\", Default" w2021 {
                      frame "X-Y-t movie", Default {
                        n5073 = local read "avpp"() -> (w2042:i32)
                        n5074 = local read "Angle ref"() -> (w2041:dbl)
                        n5075 = local read "ROI Type"() -> (w2040:u16)
                        n5076 = local read "xpixels ref"() -> (w2037:i32)
                        n5077 = local read "Vx-min ref"() -> (w2036:dbl)
                        n5078 = local read "Vx-max ref"() -> (w2035:dbl)
                        n5079 = local read "ypixels ref"() -> (w2033:i32)
                        n5080 = local read "Vy-min ref"() -> (w2034:dbl)
                        n5081 = local read "Vy-max ref"() -> (w2030:dbl)
                        n5082 = local read "Sampling rate"() -> (w2024:dbl)
                        n5083 = local read "finite samples"() -> (w2025:bool)
                        n5084 = local read "continuous"() -> (w2028:bool)
                        n5085 = local read "wavdet"() -> (w2029:bool)
                        n5086 = local read "# of frames"() -> (w2027:i32)
                        n5087 = local read "maxbufferAI"() -> (w2026:i32)
                        n5088 = local read "Override AI buffer"() -> (w2022:bool)
                        n5089 = call "2pparameters.vi"("command"="get") -> ("params out"=w2039:T12)  [unwired: 1 in]
                        n5090 = Bundle By Name(cluster=w2039, "type"="X-Y-t movie", "avpp"=w2042, "Angle Img"=w2041, "Xpixels Img"=w2037, "Vx-min Img"=w2036, "VX-max Img"=w2035, "Ypixels Img"=w2033, "Vy-min Img"=w2034, "Vy-max Img"=w2030, "srate"=w2024, "srate Img"=w2024, "finite"=w2025, "cont"=w2028, "wavdet"=w2029, "measpoints"=w2027, "maxbufferAI"=w2026, "Drawing Mode"=w2040, "Vz-reset"=0.0, "AIoverride"=w2022) -> (w2031:T12)
                        n5091 = call "2pparameters.vi"("Params in"=w2031, "command"="set") -> ()  [unwired: 1 out]
                      }
                      frame "X-Y-Z stack" {
                        n5092 = call "2pparameters.vi"("command"="get") -> ("params out"=w2046:T12)  [unwired: 1 in]
                        n5093 = Bundle By Name(cluster=w2046, "type"="X-Y-Z stack") -> (w2044:T12)
                        n5094 = call "2pparameters.vi"("Params in"=w2044, "command"="set") -> ()  [unwired: 1 out]
                      }
                      frame "Lifetime (scan)" {
                        n5095 = call "2pparameters.vi"("command"="get") -> ("params out"=w2051:T12)  [unwired: 1 in]
                        n5096 = Bundle By Name(cluster=w2051, "type"="Lifetime (scan)") -> (w2049:T12)
                        n5097 = call "2pparameters.vi"("Params in"=w2049, "command"="set") -> ()  [unwired: 1 out]
                      }
                      frame "Lifetime (contour)" {
                        n5098 = local read "Vy-min draw"() -> (w2061:dbl)
                        n5099 = local read "Vy-max draw"() -> (w2060:dbl)
                        n5100 = local read "Vx-min draw"() -> (w2063:dbl)
                        n5101 = local read "Vx-max draw"() -> (w2062:dbl)
                        n5102 = local read "xpixels ref"() -> (w2059:i32)
                        n5103 = local read "ypixels ref"() -> (w2058:i32)
                        n5104 = local read "ROI Type"() -> (w2057:u16)
                        n5105 = local read "srateAODOtt"() -> (w2068:dbl)
                        n5106 = local read "# of frames"() -> (w2073:i32)
                        n5107 = local read "refreshtime"() -> (w2065:dbl)
                        n5108 = local read "Pel"() -> (w2056:dbl)
                        n5109 = local read "bin"() -> (w2071:dbl)
                        n5110 = local read "Override AI buffer"() -> (w2054:bool)
                        n5111 = local read "finite samples"() -> (w2080:bool)
                        n5112 = local read "srateAODOtt"() -> (w2067:dbl)
                        n5113 = local read "srateAODOtt"() -> (w2074:dbl)
                        n5114 = local read "continuous"() -> (w2079:bool)
                        n5115 = local read "Angle ref"() -> (w2064:dbl)
                        n5116 = local read "wavdet"() -> (w2081:bool)
                        n5117 = local read "Vx-ref"() -> (w2076:dbl)
                        n5118 = local read "Vy-ref"() -> (w2078:dbl)
                        n5119 = local read "avpp"() -> (w2077:i32)
                        n5120 = call "tt_timeandsamples.vi"("bin"=w2071, "refreshtime"=w2065, "srateAODOtt"=w2068, "tot#ofsamples"=w2073) -> ("refreshrate"=w2069:dbl, "refreshbuffer"=w2070:i32, "timetracecycles"=w2075:i32)  [unwired: 5 in]
                        n5121 = local read "bin"() -> (w2072:dbl)
                        n5122 = call "2pparameters.vi"("command"="get") -> ("params out"=w2084:T12)  [unwired: 1 in]
                        n5123 = Bundle By Name(cluster=w2084, "Drawing Mode"=w2057, "measpoints"=w2073, "tt_cycles"=w2075, "refreshbuffer"=w2070, "refreshrate"=w2069, "Vx-ref"=w2076, "Vy-ref"=w2078, "srate"=w2067, "finite"=w2080, "cont"=w2079, "wavdet"=w2081, "avpp"=w2077, "srateAODO"=w2074, "bufferAI"=w2070, "bin"=w2072, "Angle Img"=w2064, "Vxminref"=w2063, "Vxmaxref"=w2062, "Vyminref"=w2061, "Vymaxref"=w2060, "Xpixels Img"=w2059, "Ypixels Img"=w2058, "Pel"=w2056, "Vz-reset"=0.0, "AIoverride"=w2054, "type"="Lifetime (contour)") -> (w2082:T12)
                        n5124 = Reciprocal(x=w2069) -> (1/x=w2066:dbl)
                        n5125 = local write "refreshtime"(w2066) -> ()
                        n5126 = call "2pparameters.vi"("Params in"=w2082, "command"="set") -> ()  [unwired: 1 out]
                      }
                      frame "X-Y-Z-t movie" {
                      }
                      frame "linescan" {
                      }
                      frame "Timetrace" {
                        n5127 = local read "Vy-min draw"() -> (w2094:dbl)
                        n5128 = local read "Vy-max draw"() -> (w2093:dbl)
                        n5129 = local read "Vx-min draw"() -> (w2096:dbl)
                        n5130 = local read "Vx-max draw"() -> (w2095:dbl)
                        n5131 = local read "xpixels ref"() -> (w2092:i32)
                        n5132 = local read "ypixels ref"() -> (w2091:i32)
                        n5133 = local read "ROI Type"() -> (w2090:u16)
                        n5134 = local read "srateAODOtt"() -> (w2101:dbl)
                        n5135 = local read "# of frames"() -> (w2106:i32)
                        n5136 = local read "refreshtime"() -> (w2098:dbl)
                        n5137 = local read "Pel"() -> (w2089:dbl)
                        n5138 = local read "bin"() -> (w2104:dbl)
                        n5139 = local read "Override AI buffer"() -> (w2087:bool)
                        n5140 = local read "finite samples"() -> (w2113:bool)
                        n5141 = local read "srateAODOtt"() -> (w2100:dbl)
                        n5142 = local read "srateAODOtt"() -> (w2107:dbl)
                        n5143 = local read "continuous"() -> (w2112:bool)
                        n5144 = local read "Angle ref"() -> (w2097:dbl)
                        n5145 = local read "wavdet"() -> (w2114:bool)
                        n5146 = local read "Vx-ref"() -> (w2109:dbl)
                        n5147 = local read "Vy-ref"() -> (w2111:dbl)
                        n5148 = local read "avpp"() -> (w2110:i32)
                        n5149 = call "tt_timeandsamples.vi"("bin"=w2104, "refreshtime"=w2098, "srateAODOtt"=w2101, "tot#ofsamples"=w2106) -> ("refreshrate"=w2102:dbl, "refreshbuffer"=w2103:i32, "timetracecycles"=w2108:i32)  [unwired: 5 in]
                        n5150 = local read "bin"() -> (w2105:dbl)
                        n5151 = call "2pparameters.vi"("command"="get") -> ("params out"=w2117:T12)  [unwired: 1 in]
                        n5152 = Bundle By Name(cluster=w2117, "Drawing Mode"=w2090, "measpoints"=w2106, "tt_cycles"=w2108, "refreshbuffer"=w2103, "refreshrate"=w2102, "Vx-ref"=w2109, "Vy-ref"=w2111, "srate"=w2100, "finite"=w2113, "cont"=w2112, "wavdet"=w2114, "avpp"=w2110, "srateAODO"=w2107, "bufferAI"=w2103, "bin"=w2105, "Angle Img"=w2097, "Vxminref"=w2096, "Vxmaxref"=w2095, "Vyminref"=w2094, "Vymaxref"=w2093, "Xpixels Img"=w2092, "Ypixels Img"=w2091, "Pel"=w2089, "Vz-reset"=0.0, "AIoverride"=w2087, "type"="Timetrace") -> (w2115:T12)
                        n5153 = Reciprocal(x=w2102) -> (1/x=w2099:dbl)
                        n5154 = local write "refreshtime"(w2099) -> ()
                        n5155 = call "2pparameters.vi"("Params in"=w2115, "command"="set") -> ()  [unwired: 1 out]
                      }
                      frame "Lifetime (point)" {
                      }
                    }
                  }
                  frame #1 {
                    w2120 = FALSE ("wavdet")
                    n5156 = call "2pparameters.vi"("command"="get") -> ("params out"=w2124:T12)  [unwired: 1 in]
                    n5157 = Bundle By Name(cluster=w2124, "finite"=w2120, "cont"=w2120, "wavdet"=TRUE) -> (w2121:T12)
                    n5158 = call "2pparameters.vi"("Params in"=w2121, "command"="set") -> ()  [unwired: 1 out]
                  }
                  frame #2 {
                    n5159 = property on="Loaded settings" class="Ring (strict)"() -> ("RingText.Text"=w2126:string)  [unwired: 2 in, 2 out]
                    n5160 = control-ref of="Analog Lines Plot"() -> (w2128:refnum<vi>)
                    n5161 = control-ref of="Digital Lines Plot"() -> (w2127:refnum<vi>)
                    n5162 = call "Usedlinesfromsettingsfile.vi"("sertting"=w2126) -> ("used AO names"=w2132:string[], "used AO lines"=w2131:tag[], "used DO names"=w2130:string[], "used DO lines"=w2129:tag[])
                    n5163 = call "loadAODOwfparamsfromsettingsfile.vi"("sertting"=w2126) -> ()
                    n5164 = call "prepAOWaveplot.vi"("WaveformGraph in"=w2128, "Analog Used Names"=w2132) -> ()  [unwired: 1 in]
                    n5165 = local write "Analog Used Names"(w2132) -> ()
                    n5166 = local write "Analog Used Lines"(w2131) -> ()
                    n5167 = call "prepDOWaveplot.vi"("DigitalGraph in"=w2127, "used DO names"=w2130) -> ()  [unwired: 1 in]
                    n5168 = local write "Digital Used Names"(w2130) -> ()
                    n5169 = local write "Digital Used Lines"(w2129) -> ()
                  }
                  frame #3 {
                    n5170 = call "waveformparamsv2.vi"("command"="get") -> ("Params out"=w2149:T17)  [unwired: 4 in, 2 out]
                    n5171 = Unbundle By Name(w2149) -> ("AO parameters"=w2150:T18, "DO parameters"=w2151:T20)
                    n5172 = for {
                      tunnel: w2150 -> [w2171] mode=indexing
                      tunnel: [w2169] -> w2152 mode=indexing
                      tunnel: [w2168] -> w2137 mode=indexing
                      tunnel: [w2166] -> w2140 mode=indexing
                      i -> [w2170]
                      n5173 = Unbundle By Name(w2171) -> ("AOtab"=w2172:dbl)
                      n5174 = To Long Integer(number=w2172) -> (32bit integer=w2165:i32)
                      n5175 = case shown="0, Default" w2165 {
                        tunnel: w2171 -> [_ w2183 w2185 w2187]
                        tunnel: [_ w2182 w2184 w2186] -> w2167
                        frame -1 {
                        }
                        frame 0, Default {
                          n5176 = call "generateRampedSquareWave_fromAOparameters.vi"("AO params"=w2183) -> ("Waveform"=w2182:waveform(dbl))  [unwired: 1 out]
                        }
                        frame 1 {
                          n5177 = call "generateTriWave_fromAOparameters.vi"("AO params"=w2185) -> ("Waveform"=w2184:waveform(dbl))  [unwired: 1 out]
                        }
                        frame 2 {
                          n5178 = call "matlabAOwffromparam.vi"("Cluster"=w2187) -> ("Waveform"=w2186:waveform(dbl))  [unwired: 1 out]
                        }
                      }
                      n5179 = case shown="0" w2170 {
                        tunnel: [w2177 -1] -> w2169
                        tunnel: [w2176 w2180] -> w2168
                        tunnel: w2167 -> [w2176 w2180]
                        tunnel: [w2173 -1.0] -> w2166
                        frame 0 {
